vi "Get Channels from Line.vi"(11 "Line":T1) -> (3 "Channels":refnum<class "TBM channel.lvclass">[](array[class]))   [LabVIEW 2015, in "PID Module configuration.lvclass"]
doc: "Returns an array of channels for a single line."
uses:
  PID Module configuration.lvclass
  <vilib>/NI/Tag Bus Module Framework/channel/TBM channel.lvclass
  Line.ctl
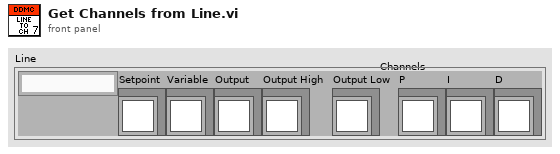
[diagram p1: front panel]
types:
  T1 = typedef "PID Module configuration.lvclass/Line.ctl" = cluster{"PID ID":string, "Setpoint":refnum<class "TBM channel.lvclass">, "Variable":refnum<class "TBM channel.lvclass">, "Output":refnum<class "TBM channel.lvclass">, "Output High":refnum<class "TBM channel.lvclass">, "Output Low":refnum<class "TBM channel.lvclass">, "P":refnum<class "TBM channel.lvclass">, "I":refnum<class "TBM channel.lvclass">, "D":refnum<class "TBM channel.lvclass">}
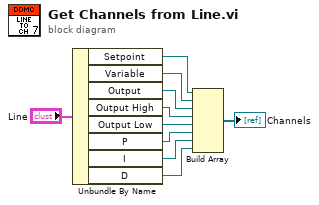
[diagram p0: block diagram]
diagram:
  n1 = Unbundle By Name("Line") -> ("Setpoint"=w8:refnum<class "TBM channel.lvclass">, "Variable"=w7:refnum<class "TBM channel.lvclass">, "Output"=w6:refnum<class "TBM channel.lvclass">, "Output High"=w5:refnum<class "TBM channel.lvclass">, "Output Low"=w4:refnum<class "TBM channel.lvclass">, "P"=w3:refnum<class "TBM channel.lvclass">, "I"=w2:refnum<class "TBM channel.lvclass">, "D"=w1:refnum<class "TBM channel.lvclass">)
  n2 = Build Array(w8, w7, w6, w5, w4, w3, w2, w1) -> (→"Channels":refnum<class "TBM channel.lvclass">[])
